vi "SolveStrive Example.vi"(8 "error in (no error)":errorcluster, 10 "ApiKey":string, 11 "Realm Id":string) -> (0 "error out":errorcluster)   [LabVIEW 2019]
uses:
  SolveStrive/control/Solvestrive Store Data.ctl
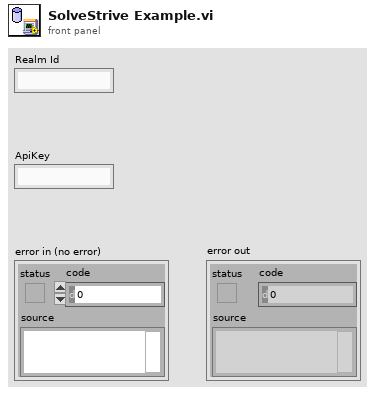
[diagram p1: front panel]
types:
  T1 = typedef "Solvestrive Store Data.ctl" = cluster{"Classification":string, "Value":dbl, "Unit":string, "timestamp":timestamp, "Realm Id":string}
  T2 = typedef "LabVIEWHTTPClient.lvlib/ClientHandle.ctl" = refnum<k1>
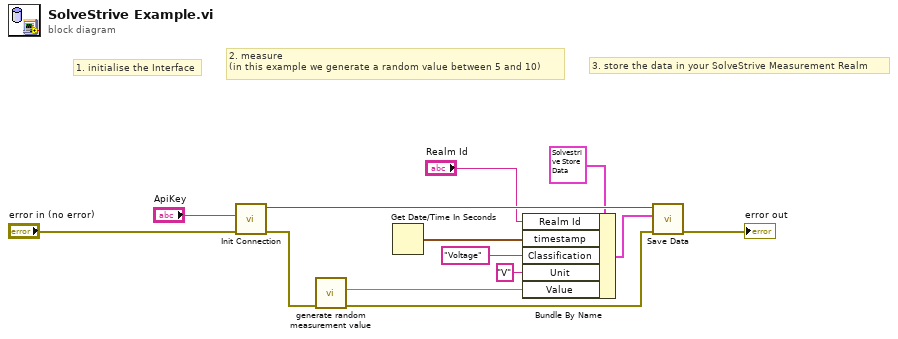
[diagram p0: block diagram]
diagram:
  # "3. store the data in your SolveStrive Measurement Realm"
  # "2. measure\n(in this example we generate a random value between 5 and 10)"
  # "1. initialise the Interface"
  n1 = call "Init Connection.vi"("error in (no error)"="error in (no error)", "ApiKey"="ApiKey") -> ("error out"=w9:errorcluster, "client handle out"=w13:T2)  [unwired: 8 in]
  n2 = call "generate random measurement value.vi"("error in (no error)"=w9) -> ("error out"=w8:errorcluster, "Random Measurement Value (5 - 10)"=w6:dbl)  [unwired: 9 in]
  n3 = Get Date/Time In Seconds() -> (seconds since 1Jan1904=w3:timestamp)
  n4 = Bundle By Name(cluster=T1 {"Classification"="", "Value"=0.0, "Unit"="", "timestamp"=timestamp(0 s since 1904-01-01), "Realm Id"=""} ("Data"), "Realm Id"="Realm Id", "timestamp"=w3, "Classification"="Voltage", "Unit"="V", "Value"=w6) -> (w7:T1)
  n5 = call "Save Data.vi"("error in (no error)"=w8, "Data"=w7, "client handle in"=w13) -> ("error out"=→"error out":errorcluster)  [unwired: 6 in, 2 out]
